vi "Configure Protection.vi"(6 "Protection (None)":T1, 8 "error in (no error)":errorcluster, 10 "Limit":dbl format="%.2f", 11 "N5745A in":refnum<class "5745A.lvclass">) -> (0 "error out":errorcluster, 3 "N5745A out":refnum<class "5745A.lvclass">)   [LabVIEW 2018, in "5745A.lvlib" / "5745A.lvclass"]
doc: "Configure Protection setting, available options:\n\n0: None\n1: Over Voltage\n2: Under Voltage\n3: Over Current\n\nDbl Precision Limit"
uses:
  5745A.lvclass
  builds/Power_Supply.lvlibp/Custom Control/Protection.ctl
  builds/Power_Supply.lvlibp/Power Supply.lvclass
  C:/Users/Ron.Dexter.LUMINARTECH/Desktop/builds/Power_Supply.lvlibp/Power Supply.lvclass
  builds/Power_Supply.lvlibp
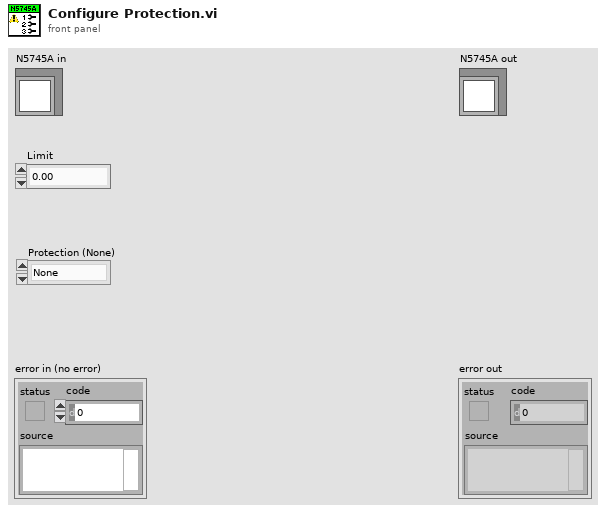
[diagram p1: front panel]
types:
  T1 = typedef "Power_Supply.lvlibp/Protection.ctl" = enum16{"None", "Over Volt", "Under Volt", "Over Current"}
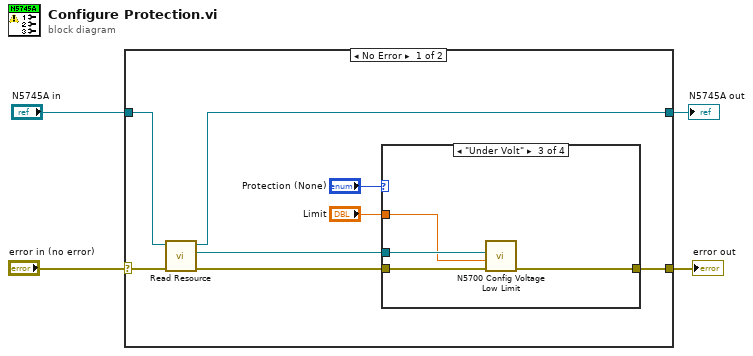
[diagram p0: block diagram]
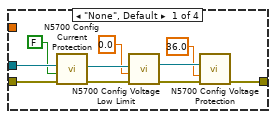
[diagram p2: hidden frame]
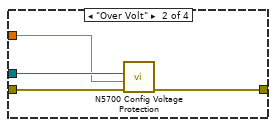
[diagram p3: hidden frame]
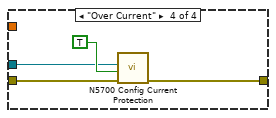
[diagram p4: hidden frame]
diagram:
  n1 = case shown="No Error" "error in (no error)" {
    selector: "error in (no error)" -> [w12 w35]
    tunnel: [w11 w35] -> w3
    tunnel: [w5 w36] -> w1
    tunnel: "N5745A in" -> [w8 w36]
    frame No Error {
      n2 = call "Read Resource.vi"("error in"=w12, "Power Supply in"=w8) -> ("error out"=w9:errorcluster, "Resource"=w7:refnum<visa-resource-name>, "Power Supply out"=w5:refnum<class "5745A.lvclass">)  [unwired: 7 in]
      n3 = case shown="\"Under Volt\"" "Protection (None)" {
        tunnel: [w17 w24 w29 w33] -> w11
        tunnel: w9 -> [w22 w25 w30 w32]
        tunnel: w7 -> [w21 w26 w28 w31]
        tunnel: "Limit" -> [_ w23 w27 _]
        frame "None", Default {
          n4 = call <instrlib>:"N5700 Config Current Protection.vi"("error"=w22, "OCP ON"=FALSE, "VISA"=w21) -> ("error out"=w19:errorcluster, "VISA out"=w16:refnum<visa-resource-name>)  [unwired: 4 in]
          n5 = call <instrlib>:"N5700 Config Voltage Low Limit.vi"("error"=w19, "UVL Level"=0.0, "VISA"=w16) -> ("error out"=w18:errorcluster, "VISA out"=w15:refnum<visa-resource-name>)  [unwired: 4 in]
          n6 = call <instrlib>:"N5700 Config Voltage Protection.vi"("error"=w18, "OVP Level"=36.0, "VISA"=w15) -> ("error out"=w17:errorcluster)  [unwired: 4 in, 1 out]
        }
        frame "Over Volt" {
          n7 = call <instrlib>:"N5700 Config Voltage Protection.vi"("error"=w25, "OVP Level"=w23, "VISA"=w26) -> ("error out"=w24:errorcluster)  [unwired: 4 in, 1 out]
        }
        frame "Under Volt" {
          n8 = call <instrlib>:"N5700 Config Voltage Low Limit.vi"("error"=w30, "UVL Level"=w27, "VISA"=w28) -> ("error out"=w29:errorcluster)  [unwired: 4 in, 1 out]
        }
        frame "Over Current" {
          n9 = call <instrlib>:"N5700 Config Current Protection.vi"("error"=w32, "OCP ON"=TRUE, "VISA"=w31) -> ("error out"=w33:errorcluster)  [unwired: 4 in, 1 out]
        }
      }
    }
    frame Error {
    }
  }
  "error out" <- w3
  "N5745A out" <- w1
